vi "readInXml.vi"(8 "error in (no error)":errorcluster, 10 "xmlString":string, 11 "XmlParser in":refnum<class "XmlParser.lvclass">) -> (0 "error out":errorcluster, 2 "xmlNode":refnum<class "xmlNode.lvclass">, 3 "XmlParser out":refnum<class "XmlParser.lvclass">)   [LabVIEW 2009, in "Tools.lvlib" / "xml.lvlib" / "XmlParser.lvclass"]
doc: "read xml string to an xml node."
uses:
  XmlParser.lvclass
  xmlNode/xmlNode.lvclass
panel:
  out "xmlString 2":string
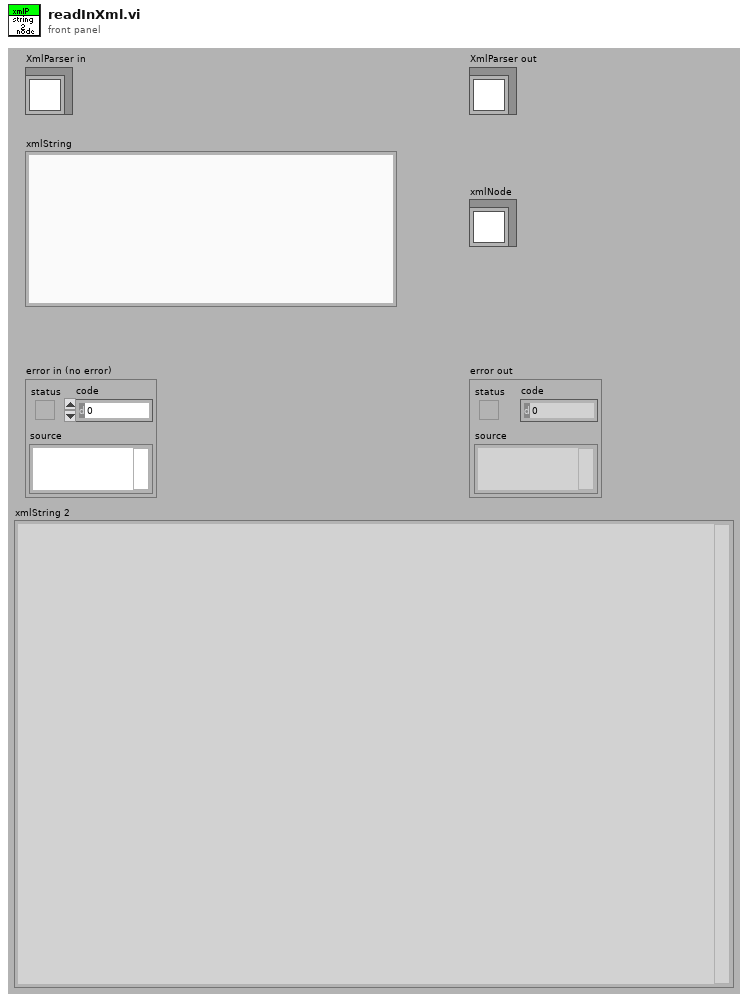
[diagram p1: front panel]
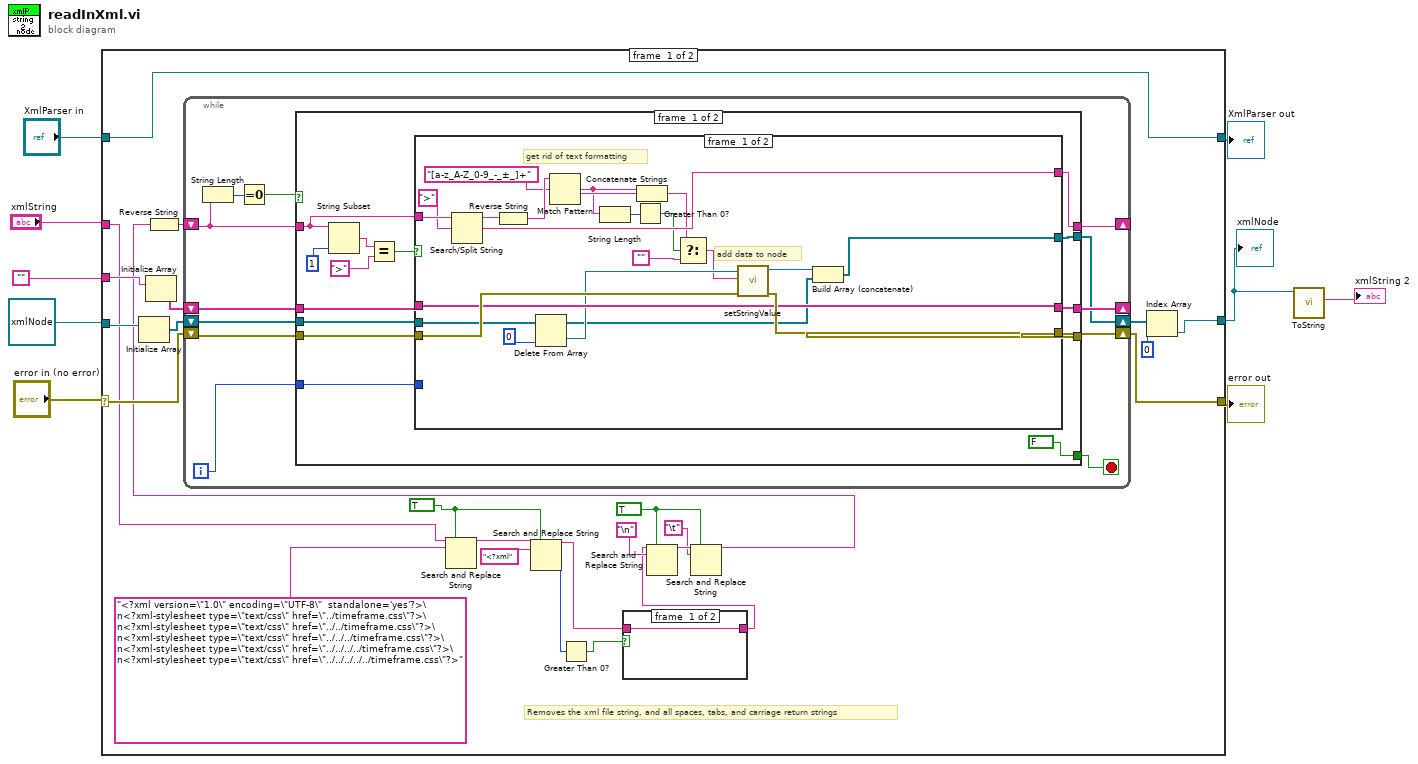
[diagram p0: block diagram]
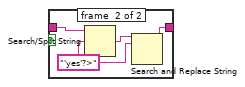
[diagram p2: hidden frame]
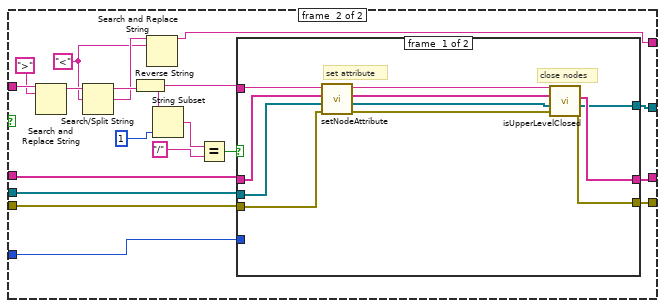
[diagram p3: hidden frame]
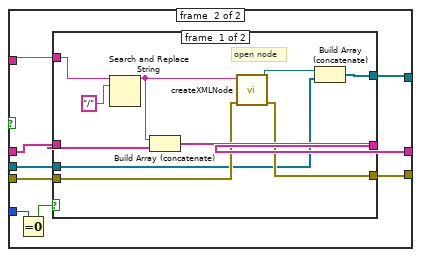
[diagram p4: hidden frame]
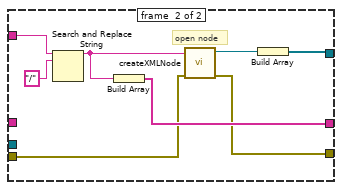
[diagram p5: hidden frame]
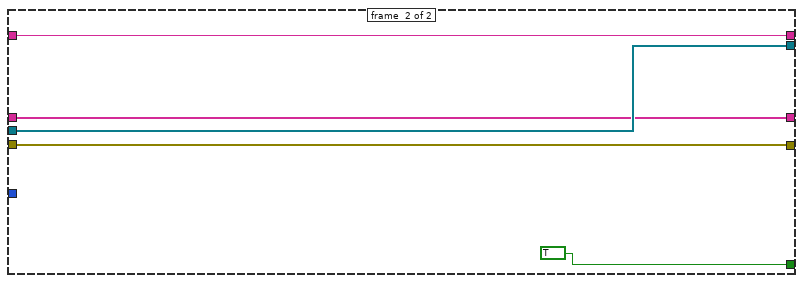
[diagram p6: hidden frame]
diagram:
  n1 = case shown="No Error" "error in (no error)" {
    selector: "error in (no error)" -> [w32 w151]
    tunnel: [w28 w151] -> w8
    tunnel: [w34 w150] -> w6
    tunnel: "XmlParser in" -> [w34 w150]
    tunnel: "xmlString" -> [w11 _]
    tunnel: [w30 _] -> w2
    tunnel: refnum<class "xmlNode.lvclass"> refnum ("Tools.lvlib:xmlNode.lvclass") -> [w21 _]
    tunnel: "" -> [w23 _]
    frame #0 {
      w13 = TRUE
      w19 = TRUE
      # "Removes the xml file string, and all spaces, tabs, and carriage return strings"
      n2 = Initialize Array(w21) -> (w22:refnum<class "xmlNode.lvclass">[])  [unwired: 1 in]
      n3 = Initialize Array(w23) -> (w24:string[])  [unwired: 1 in]
      n4 = Search and Replace String(replace all?=w13, input string=w11, search string="<?xml version=\"1.0\" encoding=\"UTF-8\"  standalone='yes'?>\n<?xml-stylesheet type=\"text/css\" href=\"../timeframe.css\"?>\n<?xml-stylesheet type=\"text/css\" href=\"../../timeframe.css\"?>\n<?xml-stylesheet type=\"text/css\" href=\"../../../timeframe.css\"?>\n<?xml-stylesheet type=\"text/css\" href=\"../../../../timeframe.css\"?>\n<?xml-stylesheet type=\"text/css\" href=\"../../../../../timeframe.css\"?>") -> (result string=w10:string)  [unwired: 5 in, 3 out]
      n5 = Search and Replace String(replace all?=w13, input string=w10, search string="<?xml") -> (result string=w17:string, number of replacements=w14:i32)  [unwired: 5 in, 2 out]
      n6 = Greater Than 0?(x=w14) -> (x > 0?=w16:bool)
      n7 = case shown="True" w16 {
        tunnel: w17 -> [w35 w39]
        tunnel: [w35 w36] -> w15
        frame #0 {
        }
        frame #1 {
          w37 = "'yes'?>"
          n8 = Search/Split String(string=w39, search string/char (-)=w37) -> (match + rest of string=w38:string)  [unwired: 1 in, 2 out]
          n9 = Search and Replace String(input string=w38, search string=w37) -> (result string=w36:string)  [unwired: 6 in, 3 out]
        }
      }
      n10 = Search and Replace String(replace all?=w19, input string=w15, search string="\n") -> (result string=w26:string)  [unwired: 5 in, 3 out]
      n11 = Search and Replace String(replace all?=w19, input string=w26, search string="\t") -> (result string=w20:string)  [unwired: 5 in, 3 out]
      n12 = Reverse String(1:w20) -> (0:w33:string)
      n13 = while {
        shift-right: [w48] -> w29
        shift-left: w22 -> [w51]
        shift-right: [w45] -> _
        shift-left: w33 -> [w41]
        shift-right: [w50] -> _
        shift-left: w24 -> [w49]
        shift-right: [w47] -> w28
        shift-left: w32 -> [w46]
        i -> [w40]
        stop <- w43 stop-if-true
        n14 = String Length(string=w41) -> (length=w44:i32)
        n15 = Equal To 0?(x=w44) -> (x = 0?=w42:bool)
        n16 = case shown="False" w42 {
          tunnel: w51 -> [w61 w148]
          tunnel: [w60 w146] -> w50
          tunnel: w49 -> [w59 w146]
          tunnel: [w58 w148] -> w48
          tunnel: [w57 w145] -> w47
          tunnel: w46 -> [w56 w145]
          tunnel: [w55 w147] -> w45
          tunnel: w41 -> [w54 w147]
          tunnel: [FALSE TRUE] -> w43
          tunnel: w40 -> [w52 _]
          frame #0 {
            n17 = String Subset(string=w54, length (rest)=1) -> (substring=w64:string)  [unwired: 1 in]
            n18 = Equal?(x=w64, y=">") -> (x = y?=w62:bool)
            n19 = case shown="True" w62 {
              tunnel: w54 -> [w87 w95]
              tunnel: w61 -> [w84 w102]
              tunnel: w56 -> [w86 w101]
              tunnel: [w82 w100] -> w60
              tunnel: w59 -> [w82 w99]
              tunnel: [w83 w98] -> w58
              tunnel: [w85 w97] -> w57
              tunnel: [w81 w89] -> w55
              tunnel: w52 -> [_ w88]
              frame #0 {
                # "get rid of text formatting"
                # "add data to node"
                n20 = Search/Split String(string=w87, search string/char (-)=">") -> (substring before match=w78:string, match + rest of string=w81:string)  [unwired: 1 in, 1 out]
                n21 = Reverse String(1:w78) -> (0:w74:string)
                n22 = Delete From Array(array=w84, index=0) -> (deleted portion=w76:refnum<class "xmlNode.lvclass">, array with subset deleted=w75:refnum<class "xmlNode.lvclass">[])  [unwired: 1 in]
                n23 = Match Pattern(string=w74, regular expression="[a-z_A-Z_0-9_-_±_]+") -> (match substring=w71:string, after substring=w72:string)  [unwired: 1 in, 2 out]
                n24 = String Length(string=w71) -> (length=w70:i32)
                n25 = Greater Than 0?(x=w70) -> (x > 0?=w69:bool)
                n26 = Concatenate Strings(w71, w72) -> (w68:string)
                n27 = Select(t=w68, s=w69, f="") -> (s? t:f=w66:string)
                n28 = call-dynamic "setStringValue.vi"("error in (no error)"=w86, "stringValue"=w66, "xmlNode.lvclass in"=w76) -> ("error out"=w85:errorcluster, "xmlNode.lvclass out"=w79:refnum<class "xmlNode.lvclass">)  [unwired: 7 in]
                n29 = Build Array (concatenate)(w79, w75) -> (w83:refnum<class "xmlNode.lvclass">[])
              }
              frame #1 {
                w90 = "<"
                n30 = Search and Replace String(input string=w95, search string=">") -> (result string=w92:string)  [unwired: 6 in, 3 out]
                n31 = Search/Split String(string=w92, search string/char (-)=w90) -> (substring before match=w93:string, match + rest of string=w91:string)  [unwired: 1 in, 1 out]
                n32 = Reverse String(1:w93) -> (0:w96:string)
                n33 = Search and Replace String(input string=w91, search string=w90) -> (result string=w89:string)  [unwired: 6 in, 3 out]
                n34 = String Subset(string=w96, length (rest)=1) -> (substring=w105:string)  [unwired: 1 in]
                n35 = Equal?(x=w105, y="/") -> (x = y?=w103:bool)
                n36 = case shown="False" w103 {
                  tunnel: w102 -> [w110 w120]
                  tunnel: w101 -> [w108 w121]
                  tunnel: w96 -> [w114 w124]
                  tunnel: [w116 w126] -> w100
                  tunnel: w99 -> [w112 w125]
                  tunnel: [w115 w118] -> w98
                  tunnel: [w117 w119] -> w97
                  tunnel: w88 -> [_ w122]
                  frame #0 {
                    # "set attribute"
                    # "close nodes"
                    n37 = call "setNodeAttribute.vi"("error in (no error)"=w108, "open nodes"=w110, "open names"=w112, "name in"=w114) -> ("error out"=w107:errorcluster, "open nodes out"=w109:refnum<class "xmlNode.lvclass">[], "open names out"=w111:string[], "name out"=w113:string)  [unwired: 4 in]
                    n38 = call "isUpperLevelClosed.vi"("error in (no error)"=w107, "open nodes"=w109, "open names"=w111, "name to close"=w113) -> ("error out"=w117:errorcluster, "open nodes out"=w115:refnum<class "xmlNode.lvclass">[], "open names out"=w116:string[])  [unwired: 5 in]
                  }
                  frame #1 {
                    n39 = Equal To 0?(x=w122) -> (x = 0?=w123:bool)
                    n40 = case shown="False" w123 {
                      tunnel: [w133 w144] -> w126
                      tunnel: w125 -> [w134 _]
                      tunnel: w124 -> [w135 w143]
                      tunnel: w121 -> [w131 w140]
                      tunnel: w120 -> [w129 _]
                      tunnel: [w130 w139] -> w119
                      tunnel: [w127 w137] -> w118
                      frame #0 {
                        # "open node"
                        n41 = Search and Replace String(input string=w135, search string="/") -> (result string=w132:string)  [unwired: 6 in, 3 out]
                        n42 = Build Array (concatenate)(w132, w134) -> (w133:string[])
                        n43 = call "createXMLNode.vi"("error in (no error)"=w131, "name"=w132) -> ("error out"=w130:errorcluster, "xmlNode out"=w128:refnum<class "xmlNode.lvclass">)  [unwired: 8 in]
                        n44 = Build Array (concatenate)(w128, w129) -> (w127:refnum<class "xmlNode.lvclass">[])
                      }
                      frame #1 {
                        # "open node"
                        n45 = Search and Replace String(input string=w143, search string="/") -> (result string=w141:string)  [unwired: 6 in, 3 out]
                        n46 = Build Array(w141) -> (w144:string[])
                        n47 = call "createXMLNode.vi"("error in (no error)"=w140, "name"=w141) -> ("error out"=w139:errorcluster, "xmlNode out"=w138:refnum<class "xmlNode.lvclass">)  [unwired: 8 in]
                        n48 = Build Array(w138) -> (w137:refnum<class "xmlNode.lvclass">[])
                      }
                    }
                  }
                }
              }
            }
          }
          frame #1 {
          }
        }
      }
      n49 = Index Array(array=w29, index=0) -> (element=w30:refnum<class "xmlNode.lvclass">)
    }
    frame #1 {
    }
  }
  "error out" <- w8
  "XmlParser out" <- w6
  "xmlNode" <- w2
  n50 = call-dynamic "ToString.vi"("xmlNode in"=w2) -> ("xml"=→"xmlString 2":string)  [unwired: 8 in, 2 out]
